vi "Separator.vi"() -> (0 "delimiter":string)   [LabVIEW 2020, in "LUnit Utilities.lvlib"]
uses:
  Result Model/Result Model.lvclass/Result Model.ctl
  LUnit Utilities.lvlib
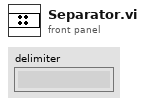
[diagram p1: front panel]
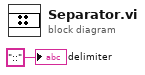
[diagram p0: block diagram]
diagram:
  "delimiter" <- "::" ("delimiter")
